vi "Read Potting Parameters.vi"(8 "error in":errorcluster, 11 "Config File Path":path) -> (0 "error out":errorcluster, 2 "Potting Parameters":T1)   [LabVIEW 2011]
uses:
  <vilib>/Utility/config.llb/Read Key (Double).vi
  <vilib>/Utility/config.llb/NI_LVConfig.lvlib
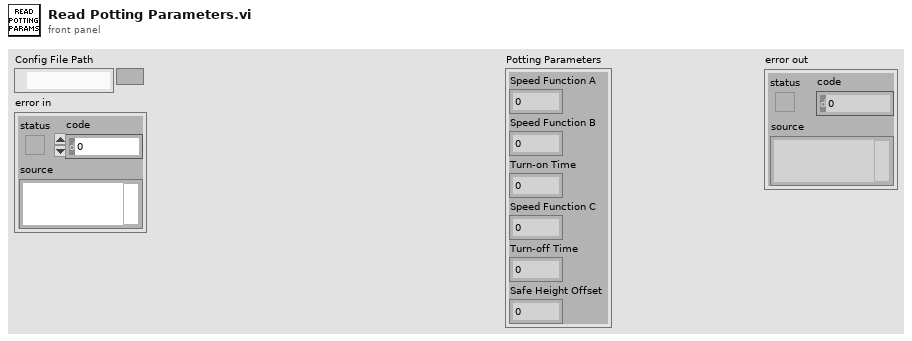
[diagram p1: front panel]
types:
  T1 = cluster{"Speed Function A":dbl, "Speed Function B":dbl, "Turn-on Time":dbl, "Speed Function C":dbl, "Turn-off Time":dbl, "Safe Height Offset":dbl}
  T2 = typedef "NI_LVConfig.lvlib/Config Data RefNum.ctl" = refnum<k1>
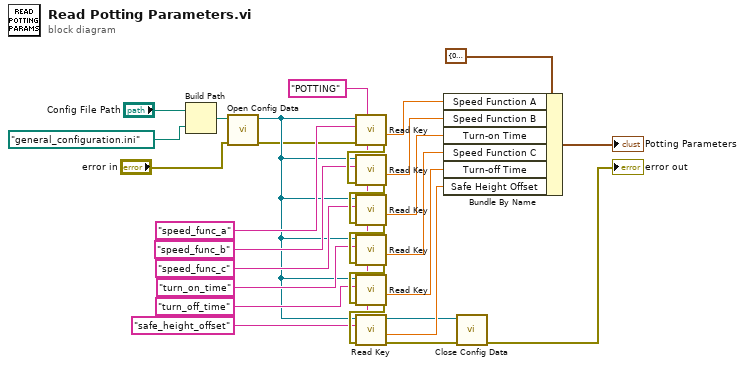
[diagram p0: block diagram]
diagram:
  w12 = "POTTING" ("section")
  n1 = Build Path(base path="Config File Path", name or relative path=path "general_configuration.ini") -> (appended path=w27:path)
  n2 = call <vilib>:"Open Config Data.vi"("error in (no error)"="error in", "configuration file path"=w27) -> ("error out"=w13:errorcluster, "refnum"=w15:T2)  [unwired: 7 in, 1 out]
  n3 = call-poly <vilib>:"Read Key.vi"("section"=w12, "error in (no error)"=w13, "key"="speed_func_a", "refnum"=w15) -> ("error out"=w26:errorcluster, "value"=w10:dbl)  [unwired: 4 in, 2 out]
  n4 = call-poly <vilib>:"Read Key.vi"("section"=w12, "error in (no error)"=w26, "key"="speed_func_b", "refnum"=w15) -> ("error out"=w25:errorcluster, "value"=w9:dbl)  [unwired: 4 in, 2 out]
  n5 = call-poly <vilib>:"Read Key.vi"("section"=w12, "error in (no error)"=w25, "key"="speed_func_c", "refnum"=w15) -> ("error out"=w24:errorcluster, "value"=w8:dbl)  [unwired: 4 in, 2 out]
  n6 = call-poly <vilib>:"Read Key.vi"("section"=w12, "error in (no error)"=w24, "key"="turn_on_time", "refnum"=w15) -> ("error out"=w23:errorcluster, "value"=w7:dbl)  [unwired: 4 in, 2 out]
  n7 = call-poly <vilib>:"Read Key.vi"("section"=w12, "error in (no error)"=w23, "key"="turn_off_time", "refnum"=w15) -> ("error out"=w22:errorcluster, "value"=w6:dbl)  [unwired: 4 in, 2 out]
  n8 = call-poly <vilib>:"Read Key.vi"("section"=w12, "error in (no error)"=w22, "key"="safe_height_offset", "refnum"=w15) -> ("error out"=w2:errorcluster, "value"=w5:dbl, "refnum out"=w3:T2)  [unwired: 4 in, 1 out]
  n9 = Bundle By Name(cluster=T1 {"Speed Function A"=0.0, "Speed Function B"=0.0, "Turn-on Time"=0.0, "Speed Function C"=0.0, "Turn-off Time"=0.0, "Safe Height Offset"=0.0}, "Speed Function A"=w10, "Speed Function B"=w9, "Turn-on Time"=w8, "Speed Function C"=w7, "Turn-off Time"=w6, "Safe Height Offset"=w5) -> (→"Potting Parameters":T1)
  n10 = call <vilib>:"Close Config Data.vi"("error in (no error)"=w2, "refnum"=w3) -> ("error out"=→"error out":errorcluster)  [unwired: 8 in, 1 out]
